vi "Master_DataStream.vi"(1 "Enum":T1=enum."Initialize", 2 "reader name in":refnum<k21>, 3 "error in":errorcluster) -> (7 "Boolean":bool, 8 "Enum out":T2=enum."Initialize", 9 "reader name out":refnum<k21>, 10 "error out":errorcluster)   [LabVIEW 2018]
doc: "Data streams for cRIO."
uses:
  Host/Libraries/TypeDef_NetworkStreamState.ctl
  Type_Def/Type_Def NetworkStreamState.ctl
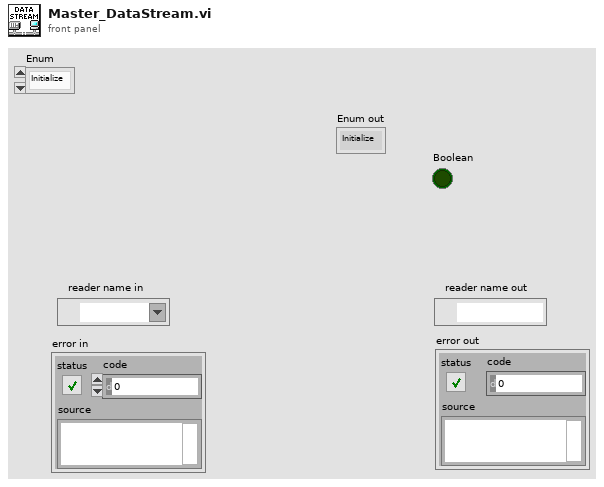
[diagram p1: front panel]
types:
  T1 = typedef "Type_Def NetworkStreamState.ctl" = enum16{"Wait", "Test", "Initialize", "Read/Write", "Terminate"}
  T2 = typedef "TypeDef_NetworkStreamState.ctl" = enum16{"Wait", "Test", "Initialize", "Read/Write", "Terminate"}
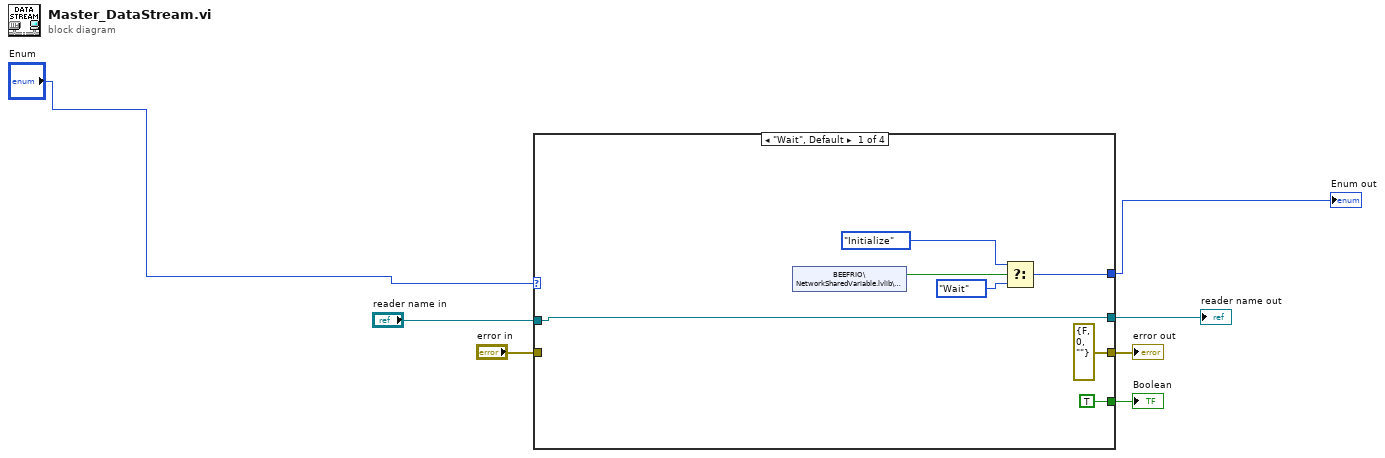
[diagram p0: block diagram]
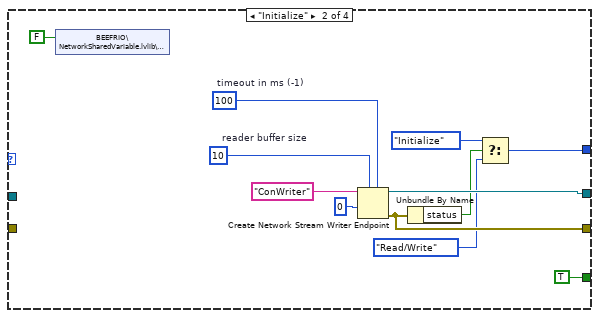
[diagram p2: hidden frame]
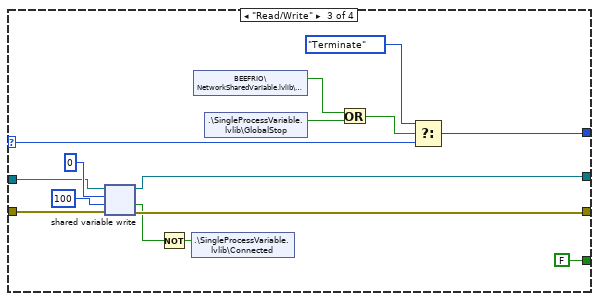
[diagram p3: hidden frame]
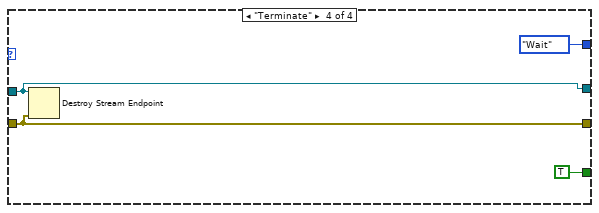
[diagram p4: hidden frame]
diagram:
  n1 = case shown="\"Wait\", Default" "Enum" {
    selector: "Enum" -> [_ _ w41 _]
    tunnel: [w14 w26 w31 w45] -> w4
    tunnel: [errorcluster {"status"=FALSE, "code"=0, "source"=""} ("error IO") w25 w32 w43] -> w7
    tunnel: "error in" -> [_ _ w30 w43]
    tunnel: "reader name in" -> [w14 _ w29 w45]
    tunnel: [w10 w21 w39 TypeDef_NetworkStreamState."Wait"] -> w2
    tunnel: [TRUE TRUE FALSE TRUE] -> w3
    frame "Wait", Default {
      n2 = shared-variable "BEEFRIO\\NetworkSharedVariable.lvlib\\ReIntStreams"() -> (w8:bool)  [unwired: 1 in, 1 out]
      n3 = Select(t=TypeDef_NetworkStreamState."Initialize", s=w8, f=TypeDef_NetworkStreamState."Wait") -> (s? t:f=w10:T2)
    }
    frame "Initialize" {
      w17 = 100  # timeout in ms (-1)
      w18 = 10  # reader buffer size
      n4 = shared-variable "BEEFRIO\\NetworkSharedVariable.lvlib\\ReIntStreams"(FALSE ("ReintStreams")) -> ()  [unwired: 1 in, 1 out]
      n5 = Create Network Stream Writer Endpoint(5:w17, 7:w18, 9:i8 0, 11:"ConWriter" ("reader name")) -> (0:w25:errorcluster, 3:w26:refnum<k21>)  [unwired: 3 in]
      n6 = Unbundle By Name(w25) -> ("status"=w24:bool)
      n7 = Select(t=TypeDef_NetworkStreamState."Initialize" ("Enum"), s=w24, f=TypeDef_NetworkStreamState."Read/Write" ("Enum")) -> (s? t:f=w21:T2)
    }
    frame "Read/Write" {
      n8 = shared-variable-write(w29, w30, i8 0, 100 ("timeout ms (-1)")) -> (w31:refnum<k21>, w32:errorcluster, w27:bool)
      n9 = Not(x=w27) -> (.not. x?=w28:bool)
      n10 = shared-variable ".\\SingleProcessVariable.lvlib\\Connected"(w28) -> ()  [unwired: 1 in, 1 out]
      n11 = shared-variable "BEEFRIO\\NetworkSharedVariable.lvlib\\ReIntStreams"() -> (w33:bool)  [unwired: 1 in, 1 out]
      n12 = shared-variable ".\\SingleProcessVariable.lvlib\\GlobalStop"() -> (w37:bool)  [unwired: 1 in, 1 out]
      n13 = Or(x=w33, y=w37) -> (x .or. y?=w38:bool)
      n14 = Select(t=TypeDef_NetworkStreamState."Terminate", s=w38, f=w41) -> (s? t:f=w39:T1)
    }
    frame "Terminate" {
      n15 = Destroy Stream Endpoint(8:w43, 11:w45) -> ()  [unwired: 1 out]
    }
  }
  "error out" <- w7
  "reader name out" <- w4
  "Boolean" <- w3
  "Enum out" <- w2
